vi "PM-filter_waveform.vi"(10 "Addition signal to remove (0) [s]":dbl, 11 "waveform in":waveform(dbl)) -> (2 "data size (s)":dbl, 3 "waveform out":waveform(dbl))   [LabVIEW 2020]
uses:
  <vilib>/Analysis/3filter.llb/Filter Passband Type.ctl
  <vilib>/Analysis/3filter.llb/Butterworth Filter (DBL).vi
  <vilib>/Analysis/NI_AALBase.lvlib
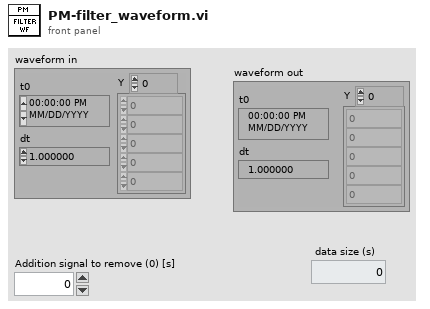
[diagram p1: front panel]
types:
  T1 = typedef "NI_AALBase.lvlib/Filter Passband Type.ctl" = enum32{"Lowpass", "Highpass", "Bandpass", "Bandstop"}
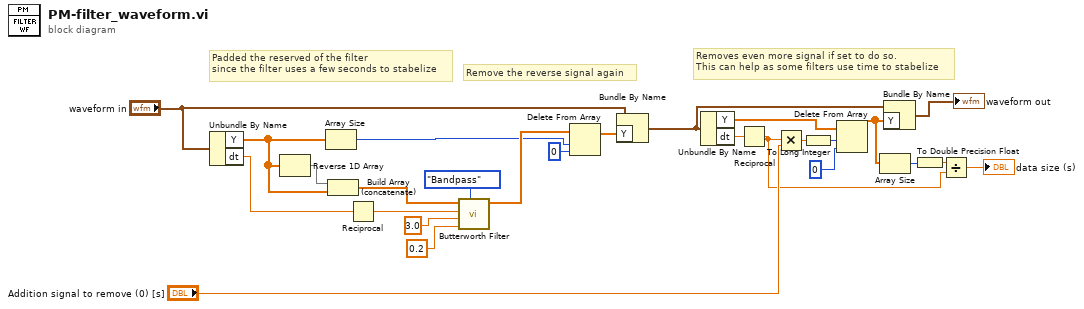
[diagram p0: block diagram]
diagram:
  # "Removes even more signal if set to do so.\nThis can help as some filters use time to stabelize"
  # "Remove the reverse signal again"
  # "Padded the reserved of the filter\nsince the filter uses a few seconds to stabelize"
  n1 = Unbundle By Name("waveform in") -> ("Y"=w1:dbl[], "dt"=w16:dbl)
  n2 = Reverse 1D Array(array=w1) -> (reversed array=w20:dbl[])
  n3 = Array Size(array=w1) -> (size(s)=w19:i32)
  n4 = Build Array (concatenate)(w20, w1) -> (w23:dbl[])
  n5 = Reciprocal(x=w16) -> (1/x=w15:dbl)
  n6 = call-poly <vilib>:"Butterworth Filter.vi"("filter type"=Filter_Passband_Type."Bandpass", "low cutoff freq: fl"=0.2, "high cutoff freq: fh"=3.0, "sampling freq: fs"=w15, "X"=w23) -> ("Filtered X"=w22:dbl[])  [unwired: 3 in, 1 out]
  n7 = Delete From Array(array=w22, length=w19, index=0) -> (array with subset deleted=w17:dbl[])  [unwired: 1 out]
  n8 = Bundle By Name(cluster="waveform in", "Y"=w17) -> (w12:waveform(dbl))
  n9 = Unbundle By Name(w12) -> ("Y"=w11:dbl[], "dt"=w10:dbl)
  n10 = Reciprocal(x=w10) -> (1/x=w2:dbl)
  n11 = Multiply(x=w2, y="Addition signal to remove (0) [s]") -> (x*y=w4:dbl)
  n12 = To Long Integer(number=w4) -> (32bit integer=w8:i32)
  n13 = Delete From Array(array=w11, length=w8, index=0) -> (array with subset deleted=w7:dbl[])  [unwired: 1 out]
  n14 = Array Size(array=w7) -> (size(s)=w6:i32)
  n15 = Bundle By Name(cluster=w12, "Y"=w7) -> (→"waveform out":waveform(dbl))
  n16 = To Double Precision Float(number=w6) -> (double precision float=w5:dbl)
  n17 = Divide(x=w5, y=w2) -> (x/y=→"data size (s)":dbl)
